vi "OE1022D_Configure_Channel_Out.vi"(0 "VISA resource name":refnum<visa-resource-name>, 1 "CH1 Offset(%)":dbl format="%.2f", 2 "CH1 Expand":dbl, 3 "CH1 Speed":u16(ring) items=["Slow", "Fast"], 5 "CH 1":u16(ring) items=["A-R", "A-X", "A-Y", "A-Theta", "A-Rh1", "A-Xh1", "A-Yh1", "A-Theta h1", "A-Rh2", "A-Xh2", "A-Yh2", "A-Theta h2", "A-Noise", "A-E1", "A-E2", "A-E3", "A-E4", "B-R", "B-X", "B-Y", "B-Theta", "B-Rh1", "B-Xh1", "B-Yh1", "B-Theta h1", "B-Rh2", "B-Xh2", "B-Yh2", "B-Theta h2", "B-Noise", "B-E1", "B-E2", "B-E3", "B-E4"], 9 "CH 2":u16(ring) items=["A-R", "A-X", "A-Y", "A-Theta", "A-Rh1", "A-Xh1", "A-Yh1", "A-Theta h1", "A-Rh2", "A-Xh2", "A-Yh2", "A-Theta h2", "A-Noise", "A-E1", "A-E2", "A-E3", "A-E4", "B-R", "B-X", "B-Y", "B-Theta", "B-Rh1", "B-Xh1", "B-Yh1", "B-Theta h1", "B-Rh2", "B-Xh2", "B-Yh2", "B-Theta h2", "B-Noise", "B-E1", "B-E2", "B-E3", "B-E4"], 11 "error in (no error)":errorcluster, 12 "CH2 Offset(%)":dbl format="%.2f", 13 "CH2 Expand":dbl, 14 "CH2 Speed":u16(ring) items=["Slow", "Fast"]) -> (4 "VISA resource name out":refnum<visa-resource-name>, 15 "error out":errorcluster)   [LabVIEW 2021]
panel:
  out "连接的字符串":string
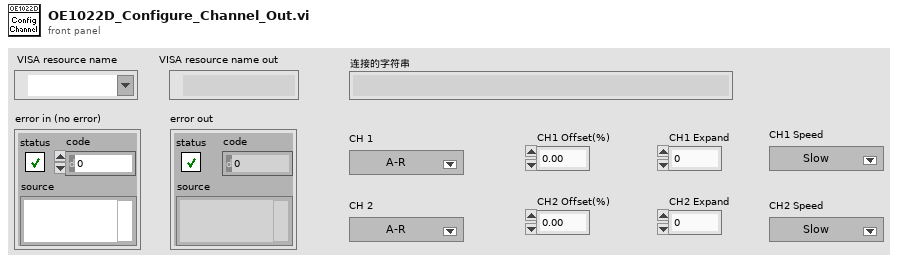
[diagram p1: front panel]
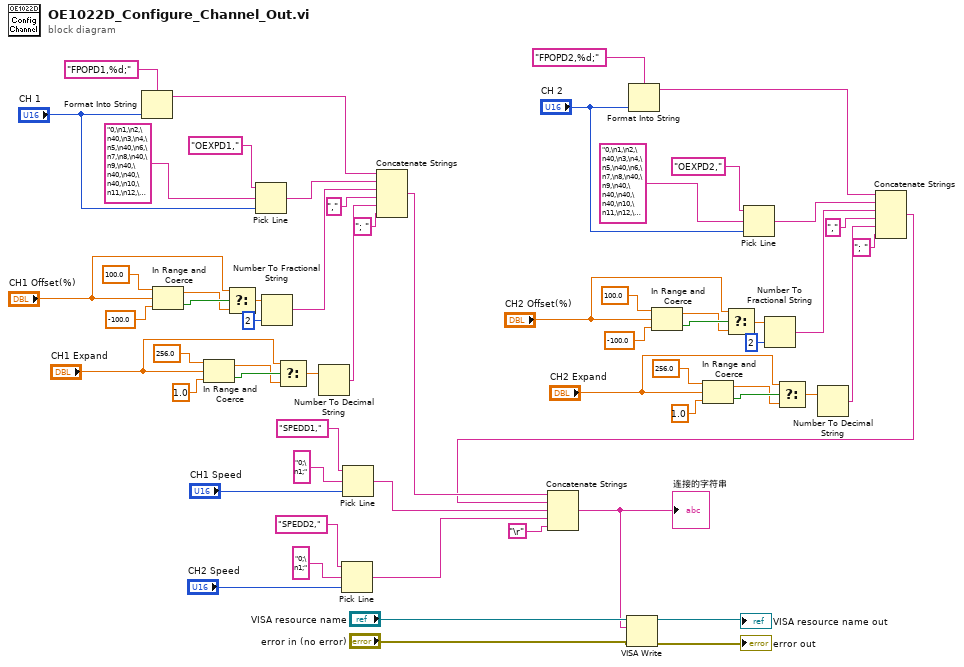
[diagram p0: block diagram]
diagram:
  n1 = Format Into String(format string="FPOPD1,%d;" ("字符串"), "CH 1") -> (resulting string=w32:string)  [unwired: 2 in, 1 out]
  n2 = In Range and Coerce(upper limit=100.0 ("上限"), x="CH1 Offset(%)", lower limit=-100.0 ("下限")) -> (coerced(x)=w54:dbl, In Range?=w56:bool)
  n3 = In Range and Coerce(upper limit=256.0 ("上限"), x="CH1 Expand", lower limit=1.0 ("下限")) -> (coerced(x)=w50:dbl, In Range?=w51:bool)
  n4 = Select(t="CH1 Offset(%)", s=w56, f=w54) -> (s? t:f=w41:dbl)
  n5 = Pick Line(string ("")="OEXPD1," ("字符串"), multi-line string="0,\n1,\n2,\n40,\n3,\n4,\n5,\n40,\n6,\n7,\n8,\n40,\n9,\n40,\n40,\n40,\n40,\n10,\n11,\n12,\n40,\n13,\n14,\n15,\n40,\n16,\n17,\n18,\n40,\n19,\n40,\n40,\n40,\n40," ("多行字符串"), line index="CH 1") -> (output string=w37:string)
  n6 = Number To Fractional String(number=w41, precision (6)=i16 2 ("精度(6)")) -> (F-format string=w40:string)  [unwired: 2 in]
  n7 = Select(t="CH1 Expand", s=w51, f=w50) -> (s? t:f=w48:dbl)
  n8 = Number To Decimal String(number=w48) -> (decimal integer string=w46:string)  [unwired: 1 in]
  n9 = Pick Line(string ("")="SPEDD2," ("字符串"), multi-line string="0;\n1;" ("多行字符串"), line index="CH2 Speed") -> (output string=w21:string)
  n10 = Pick Line(string ("")="SPEDD1," ("字符串"), multi-line string="0;\n1;" ("多行字符串"), line index="CH1 Speed") -> (output string=w28:string)
  n11 = Concatenate Strings(w32, w37, w40, ",", w46, "; " ("字符串")) -> (w44:string)
  n12 = Format Into String(format string="FPOPD2,%d;" ("字符串"), "CH 2") -> (resulting string=w35:string)  [unwired: 2 in, 1 out]
  n13 = In Range and Coerce(upper limit=100.0 ("上限"), x="CH2 Offset(%)", lower limit=-100.0 ("下限")) -> (coerced(x)=w16:dbl, In Range?=w18:bool)
  n14 = In Range and Coerce(upper limit=256.0 ("上限"), x="CH2 Expand", lower limit=1.0 ("下限")) -> (coerced(x)=w12:dbl, In Range?=w13:bool)
  n15 = Select(t="CH2 Offset(%)", s=w18, f=w16) -> (s? t:f=w5:dbl)
  n16 = Pick Line(string ("")="OEXPD2," ("字符串"), multi-line string="0,\n1,\n2,\n40,\n3,\n4,\n5,\n40,\n6,\n7,\n8,\n40,\n9,\n40,\n40,\n40,\n40,\n10,\n11,\n12,\n40,\n13,\n14,\n15,\n40,\n16,\n17,\n18,\n40,\n19,\n40,\n40,\n40,\n40," ("多行字符串"), line index="CH 2") -> (output string=w2:string)
  n17 = Number To Fractional String(number=w5, precision (6)=i16 2 ("精度(6)")) -> (F-format string=w4:string)  [unwired: 2 in]
  n18 = Select(t="CH2 Expand", s=w13, f=w12) -> (s? t:f=w10:dbl)
  n19 = Number To Decimal String(number=w10) -> (decimal integer string=w8:string)  [unwired: 1 in]
  n20 = Concatenate Strings(w35, w2, w4, ",", w8, "; " ("字符串")) -> (w43:string)
  n21 = Concatenate Strings(w44, w43, w28, w21, "\r") -> (w42:string)
  "连接的字符串" <- w42
  n22 = VISA Write(VISA resource name="VISA resource name", write buffer=w42, error in (no error)="error in (no error)") -> (VISA resource name out=→"VISA resource name out":refnum<visa-resource-name>, error out=→"error out":errorcluster)  [unwired: 1 out]
